vi "DataLog Find Tag In List.vi"(0 "may not exist (false)":bool, 5 "tag":string, 7 "tag config list in":T1[](array[typedef]) {"logging parameters" format="%.2e"; "precision" items=["0", "1", "2", "3", "4", "5", "6", "7", "8", "9", "10", "11", "12", "13", "14", "15", "16", "17"]; "limit delay" format="%.2e"; "deadband" format="%.2e"}, 11 "error in (no error)":errorcluster) -> (4 "tag config out":T1 {"logging parameters" format="%.2e"; "precision" items=["0", "1", "2", "3", "4", "5", "6", "7", "8", "9", "10", "11", "12", "13", "14", "15", "16", "17"]; "limit delay" format="%.2e"; "deadband" format="%.2e"}, 8 "tag config list out":T1[](array[typedef]) {"logging parameters" format="%.2e"; "precision" items=["0", "1", "2", "3", "4", "5", "6", "7", "8", "9", "10", "11", "12", "13", "14", "15", "16", "17"]; "limit delay" format="%.2e"; "deadband" format="%.2e"}, 10 "tag index":i32, 15 "error out":errorcluster)   [LabVIEW 2012]
doc: "Searches for a tag in the provided tag info list and returns the index in the list as well as the tag's info. When the data logging is active, the tag hash should be used so as to perform the index lookup much more efficiently."
uses:
  typedefs/clusters/t_DataLog Tag Config.ctl
  typedefs/t_DataLog Temporal Types.ctl
  typedefs/t_DataLog Value Types.ctl
  typedefs/t_DataLog Numerical Format.ctl
  typedefs/t_DataLog Logging Algorithms.ctl
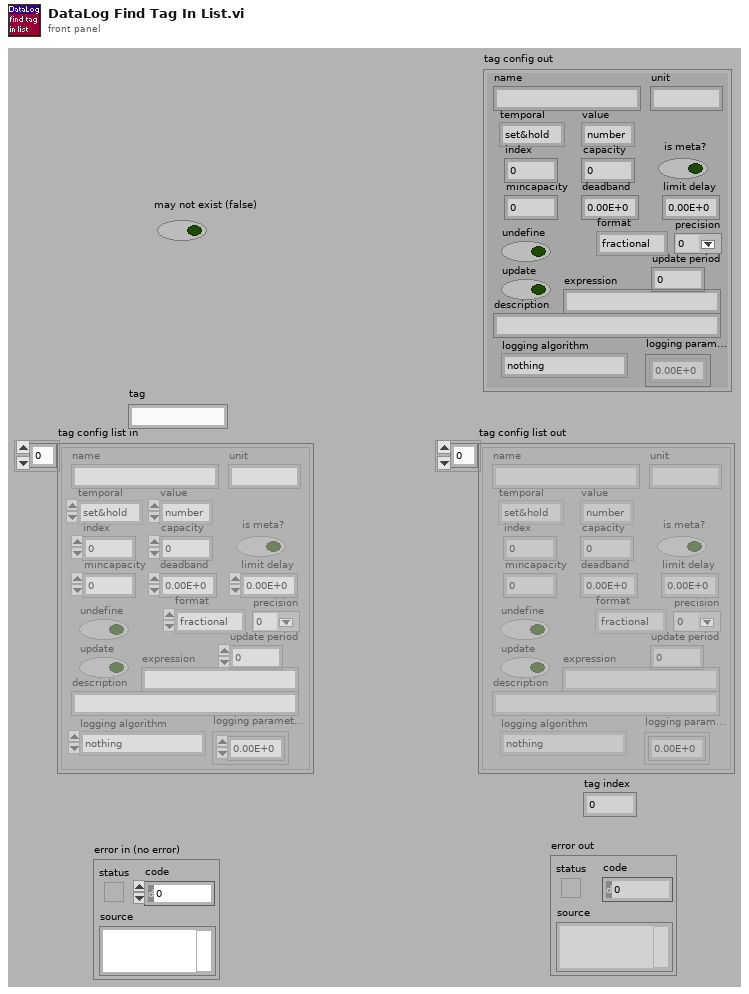
[diagram p1: front panel]
types:
  T1 = typedef "t_DataLog Tag Config.ctl" = cluster{"name":string, "unit":string, "temporal":T2, "value":T3, "index":i32, "capacity":i32, "is meta?":bool, "mincapacity":i32, "deadband":dbl, "limit delay":dbl, "format":T4, "precision":u8, "undefine":bool, "update":bool, "update period":u16, "expression":string, "description":string, "logging algorithm":T5, "logging parameters":dbl[]}
  T2 = typedef "t_DataLog Temporal Types.ctl" = enum16{"set&hold", "sample", "event"}
  T3 = typedef "t_DataLog Value Types.ctl" = enum16{"number", "string"}
  T4 = typedef "t_DataLog Numerical Format.ctl" = enum8{"fractional", "exponential", "engineering"}
  T5 = typedef "t_DataLog Logging Algorithms.ctl" = enum16{"nothing", "changes", "everything", "every Nth", "time threshold", "value threshold + prior", "t or v threshold", "t or v threshold + prior"}
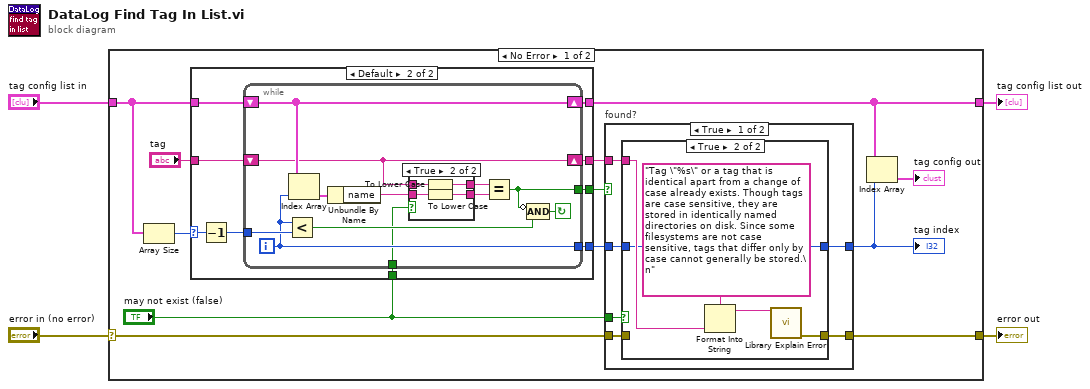
[diagram p0: block diagram]
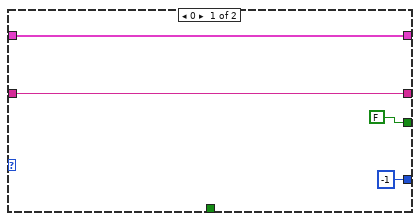
[diagram p2: hidden frame]
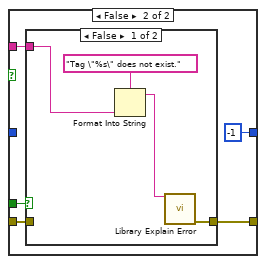
[diagram p5: hidden frame]
diagram:
  n1 = case shown="No Error" "error in (no error)" {
    selector: "error in (no error)" -> [w10 w72]
    tunnel: [w7 w71] -> w4
    tunnel: "tag config list in" -> [w16 w71]
    tunnel: [w13 w72] -> w1
    frame No Error {
      n2 = Array Size(array=w16) -> (size(s)=w9:i32)
      n3 = case shown="Default" w9 {
        selector: w9 -> [_ w22]
        tunnel: [w20 w29] -> w7
        tunnel: w16 -> [w20 w28]
        tunnel: [FALSE w26] -> w15
        tunnel: [-1 w25] -> w14
        tunnel: "tag" -> [w19 w24]
        tunnel: [w19 w23] -> w11
        tunnel: "may not exist (false)" -> [_ w21]
        frame 0 {
        }
        frame Default {
          n4 = Decrement(x=w22) -> (x-1=w27:i32)
          n5 = while {
            shift-right: [w41] -> w29
            shift-left: w28 -> [w41]
            tunnel: w27 -> [w39]
            tunnel: [w35] -> w26
            tunnel: [w34] -> w25
            shift-right: [w33] -> w23
            shift-left: w24 -> [w33]
            tunnel: w21 -> [w30]
            i -> [w34]
            stop <- w36 continue-if-true
            n6 = Less?(x=w34, y=w39) -> (x < y?=w37:bool)
            n7 = Index Array(array=w41, index=w34) -> (element=w40:T1)
            n8 = Unbundle By Name(w40) -> ("name"=w38:string)
            n9 = case shown="True" w30 {
              tunnel: w38 -> [w42 w47]
              tunnel: w33 -> [w43 w46]
              tunnel: [w43 w45] -> w32
              tunnel: [w42 w44] -> w31
              frame False {
              }
              frame True {
                n10 = To Lower Case(string=w46) -> (all lower case string=w45:string)
                n11 = To Lower Case(string=w47) -> (all lower case string=w44:string)
              }
            }
            n12 = Equal?(x=w32, y=w31) -> (x = y?=w35:bool)
            n13 = Compound Arithmetic op=AND(invert w35, w37) -> (w36:bool)
          }
        }
      }
      n14 = case "found?" shown="True" w15 {
        tunnel: w14 -> [w51 _]
        tunnel: [w50 -1 ("tag index")] -> w8
        tunnel: [w53 w65] -> w13
        tunnel: w11 -> [w52 w64]
        tunnel: w10 -> [w49 w63]
        tunnel: "may not exist (false)" -> [w48 w62]
        frame True {
          n15 = case shown="True" w48 {
            tunnel: [w54 w60] -> w53
            tunnel: w52 -> [_ w58]
            tunnel: w51 -> [w55 w56]
            tunnel: [w55 w56] -> w50
            tunnel: w49 -> [w54 _]
            frame False {
            }
            frame True {
              n16 = Format Into String(format string="Tag \"%s\" or a tag that is identical apart from a change of case already exists. Though tags are case sensitive, they are stored in identically named directories on disk. Since some filesystems are not case sensitive, tags that differ only by case cannot generally be stored.\n", w58) -> (resulting string=w57:string)  [unwired: 2 in, 1 out]
              n17 = call "Library Explain Error.vi"("explanation prefix (none)"=w57) -> ("explained error"=w60:errorcluster)  [unwired: 14 in]
            }
          }
        }
        frame False {
          n18 = case shown="False" w62 {
            tunnel: [w69 w70] -> w65
            tunnel: w64 -> [w67 _]
            tunnel: w63 -> [_ w70]
            frame False {
              n19 = Format Into String(format string="Tag \"%s\" does not exist.", w67) -> (resulting string=w66:string)  [unwired: 2 in, 1 out]
              n20 = call "Library Explain Error.vi"("explanation prefix (none)"=w66) -> ("explained error"=w69:errorcluster)  [unwired: 14 in]
            }
            frame True {
            }
          }
        }
      }
      "tag index" <- w8
      n21 = Index Array(array=w7, index=w8) -> (element=→"tag config out":T1)
    }
    frame Error {
    }
  }
  "tag config list out" <- w4
  "error out" <- w1
